vi "CRYGet Default Hardware.vi"(0 "Hardware Cluster In":T1={"Name"="", "Analog I/O"=0, "Digital I/O"=0, "Channels"=2, "Dig Dev ID"=1, "N ports"=3, "Interface"=0, "Dig I/O Ports"=[{"port #"=1, "width"=8, "direction"=0}, {"port #"=2, "width"=8, "direction"=0}, {"port #"=3, "width"=8, "direction"=0}], "Interf settings"=[], "N interfs"=3, "udev SNs"=[], "udev enable"=FALSE, "Channel Array"=[], "Cal sequence"="", "SelectedIn"=0, "SelectedOut"=0, "SelectedTab"=0, "State"=FALSE, "Help"="", "Advanced"=FALSE, "In Audio Driver"=0, "Out Audio Driver"=0} {"Channel Array"."Coupling" items=["Default"=-1, "RSE"=10083, "NRSE"=10078, "Differential"=10106, "Pseudodifferential"=12529]; "Channel Array"."term config" items=["Default"=-1, "RSE"=10083, "NRSE"=10078, "Differential"=10106, "Pseudodifferential"=12529]; "Channel Array"."Anti-aliasing Factor (%fs)" format="%.2f"}) -> (6 "I_Name Out":string[][](array[string]), 8 "O_Name Out":string[][](array[string]), 9 "Hardware Cluster Out":T1={"Name"="", "Analog I/O"=0, "Digital I/O"=0, "Channels"=2, "Dig Dev ID"=1, "N ports"=3, "Interface"=0, "Dig I/O Ports"=[{"port #"=1, "width"=8, "direction"=0}, {"port #"=2, "width"=8, "direction"=0}, {"port #"=3, "width"=8, "direction"=0}], "Interf settings"=[], "N interfs"=3, "udev SNs"=[], "udev enable"=FALSE, "Channel Array"=[], "Cal sequence"="", "SelectedIn"=0, "SelectedOut"=0, "SelectedTab"=0, "State"=FALSE, "Help"="", "Advanced"=FALSE, "In Audio Driver"=0, "Out Audio Driver"=0} {"Channel Array"."Coupling" items=["Default"=-1, "RSE"=10083, "NRSE"=10078, "Differential"=10106, "Pseudodifferential"=12529]; "Channel Array"."term config" items=["Default"=-1, "RSE"=10083, "NRSE"=10078, "Differential"=10106, "Pseudodifferential"=12529]; "Channel Array"."Anti-aliasing Factor (%fs)" format="%.2f"}, 10 "O_Device Info Out":T3(array[cluster]), 11 "AO_Hardware Channel Name Out":string[](array[string]), 12 "I_Device Info Out":T3(array[cluster]), 13 "AI_Hardware Channel Name Out":string[](array[string]), 14 "O_Channel Info Out":T2[](array[typedef]) {"Coupling" items=["Default"=-1, "RSE"=10083, "NRSE"=10078, "Differential"=10106, "Pseudodifferential"=12529]; "term config" items=["Default"=-1, "RSE"=10083, "NRSE"=10078, "Differential"=10106, "Pseudodifferential"=12529]; "Anti-aliasing Factor (%fs)" format="%.2f"}, 15 "I_Channel Info Out":T2[](array[typedef]) {"Coupling" items=["Default"=-1, "RSE"=10083, "NRSE"=10078, "Differential"=10106, "Pseudodifferential"=12529]; "term config" items=["Default"=-1, "RSE"=10083, "NRSE"=10078, "Differential"=10106, "Pseudodifferential"=12529]; "Anti-aliasing Factor (%fs)" format="%.2f"}, 16 "Real Output Device Name Out":cluster{"MME":string[], "ASIO":string[]}, 17 "Real Input Device Name Out":cluster{"MME":string[], "ASIO":string[]}, 18 "Error":bool, 19 "No Device Name":string[](array[string]))   [LabVIEW 2013]
uses:
  Typedef Control/CRYHardware Channel Info.ctl
  Typedef Control/CRYHardware.ctl
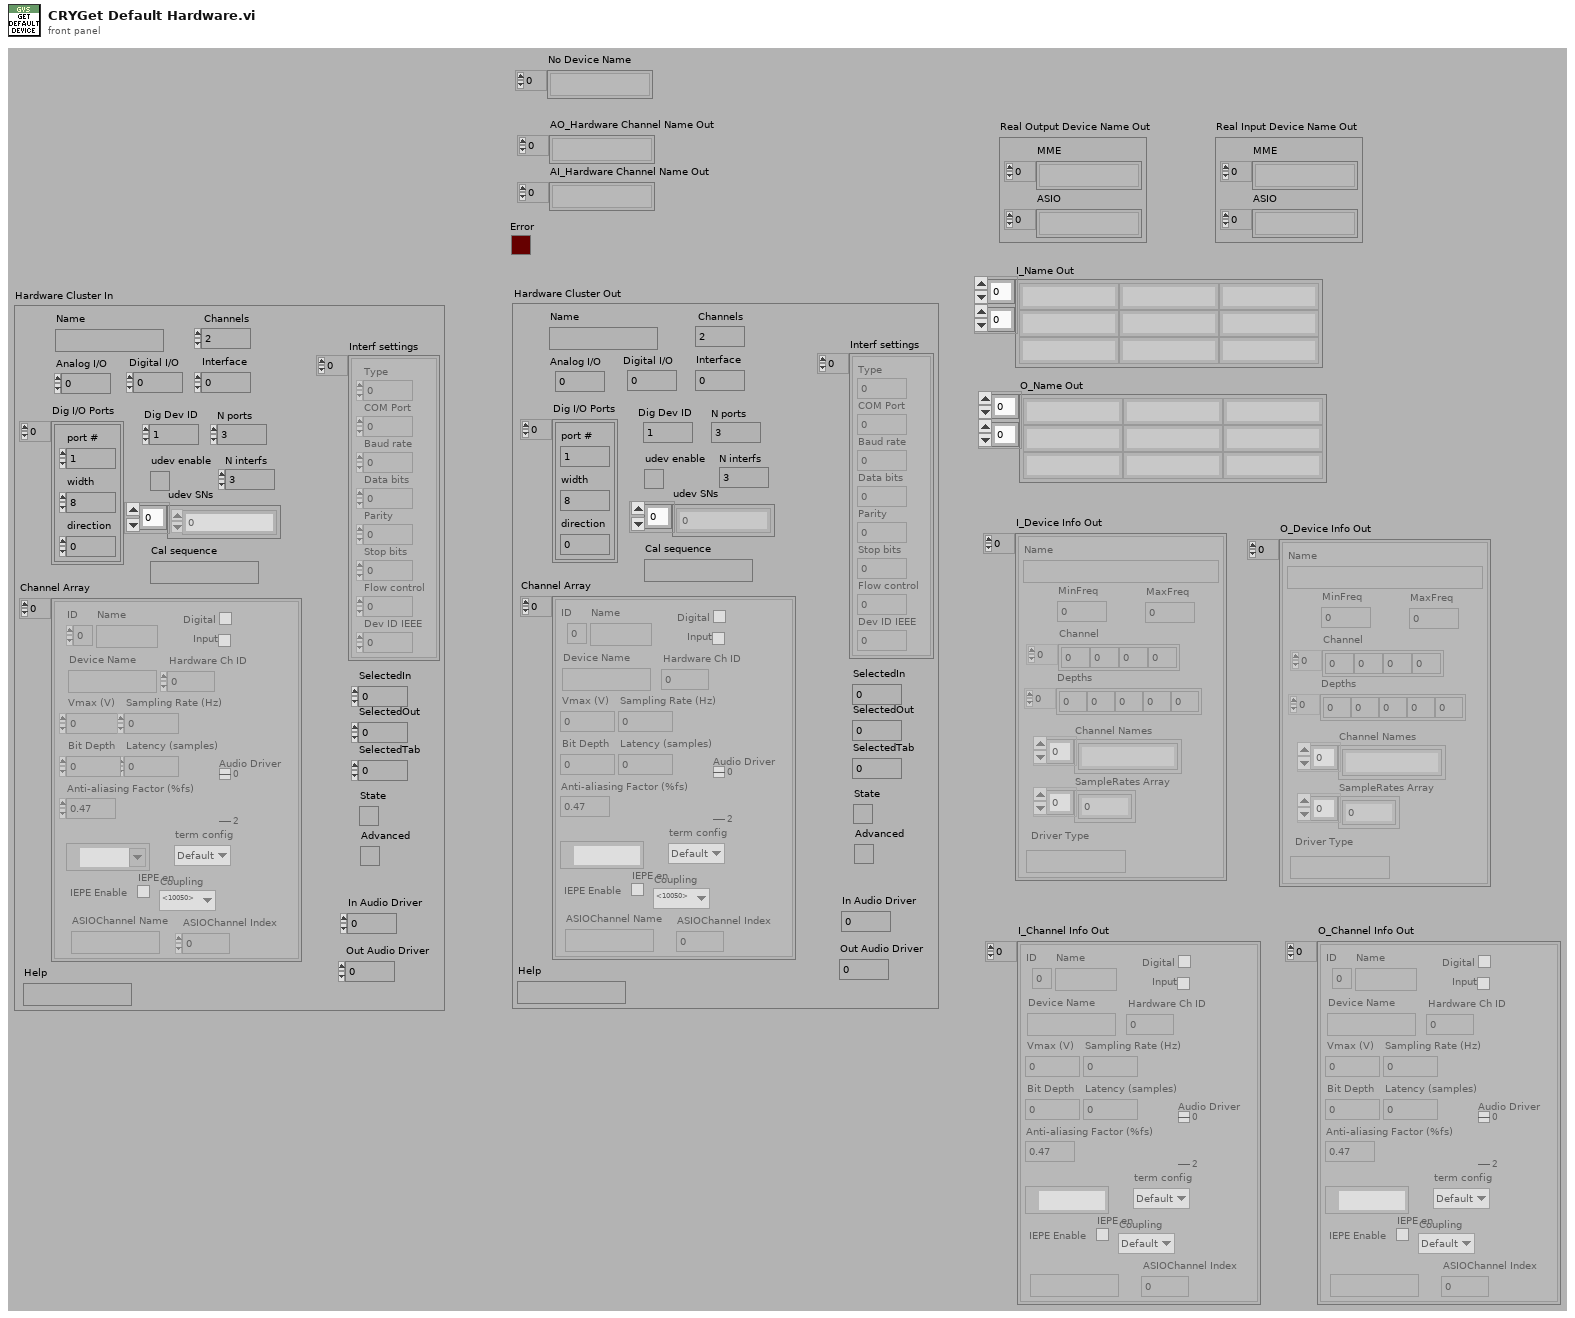
[diagram p1: front panel]
types:
  T1 = typedef "CRYHardware.ctl" = cluster{"Name":string, "Analog I/O":u16, "Digital I/O":u16, "Channels":u8, "Dig Dev ID":u8, "N ports":u8, "Interface":u32, "Dig I/O Ports":cluster{"port #":i16, "width":i16, "direction":i32}[], "Interf settings":cluster{"Type":u16, "COM Port":u8, "Baud rate":u32, "Data bits":u32, "Parity":u16, "Stop bits":u16, "Flow control":u16, "Dev ID IEEE":u8}[], "N interfs":i32, "udev SNs":i16[], "udev enable":bool, "Channel Array":T2[], "Cal sequence":string, "SelectedIn":u16, "SelectedOut":u16, "SelectedTab":u16, "State":bool, "Help":string, "Advanced":bool, "In Audio Driver":u16, "Out Audio Driver":u16}
  T2 = typedef "CRYHardware Channel Info.ctl" = cluster{"ID":i32, "Name":string, "Digital":bool, "Input":bool, "Device Name":string, "Hardware Ch ID":u8, "Vmax (V)":dbl, "Latency (samples)":dbl, "Sampling Rate (Hz)":u32, "Bit Depth":u32, "Anti-aliasing Factor (%fs)":sgl, "DAQmx Channel":tag, "term config":i32, "Coupling":i32, "IEPE en":bool, "ASIOChannel Name":string, "Audio Driver":u16, "ASIOChannel Index":u8}
  T3 = cluster{"Name":string, "MinFreq":dbl, "MaxFreq":dbl, "Channel":i32[], "Depths":i32[], "Channel Names":string[], "SampleRates Array":dbl[], "Driver Type":string}[]
  T4 = cluster{"Type":u16, "COM Port":u8, "Baud rate":u32, "Data bits":u32, "Parity":u16, "Stop bits":u16, "Flow control":u16, "Dev ID IEEE":u8}[]
  T5 = cluster{"port #":i16, "width":i16, "direction":i32}[]
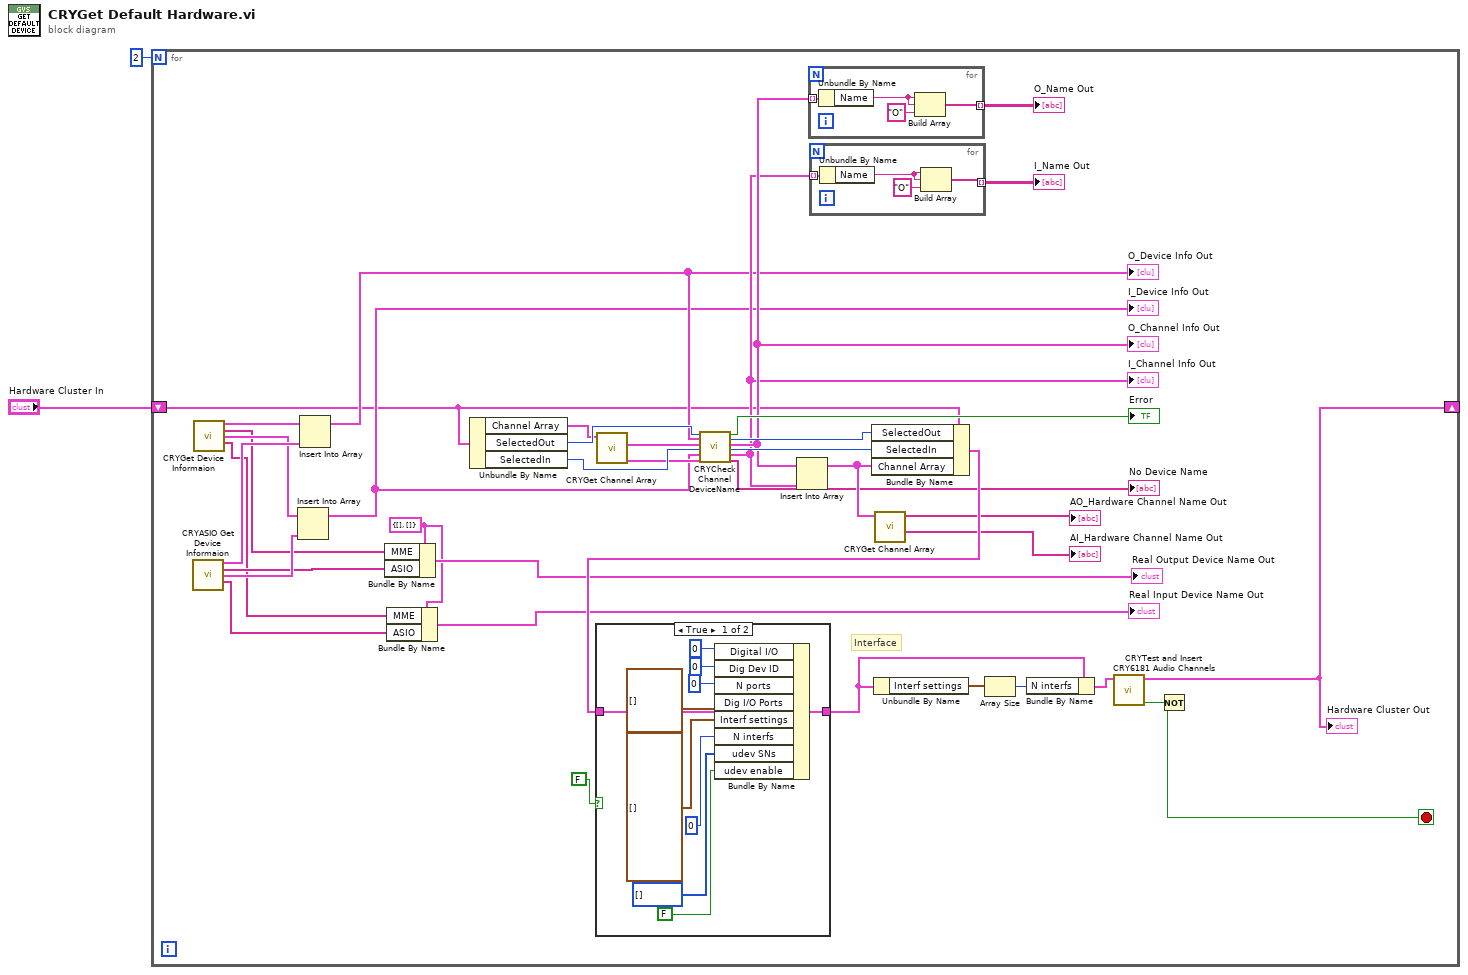
[diagram p0: block diagram]
diagram:
  n1 = for {
    N: 2 -> [_]
    shift-right: [w5] -> _
    shift-left: "Hardware Cluster In" -> [w9]
    stop <- w6 stop-if-true
    w13 = cluster{"MME":string[], "ASIO":string[]} {"MME"=[], "ASIO"=[]} ("Output Device Name Out")
    # "Interface"
    n2 = call "CRYASIO Get Device Informaion.vi"() -> ("ASIO Output Device Infor"=w22:T3, "ASIO Output Device Name"=w15:string[], "ASIO Input Device Infor"=w18:T3, "ASIO Input Device Name"=w10:string[])  [unwired: 11 in, 1 out]
    n3 = call "CRYGet Device Informaion.vi"() -> ("Output Device Infor"=w21:T3, "Output Device Name"=w16:string[], "Input Device Infor"=w19:T3, "Input Device Name"=w11:string[])  [unwired: 11 in, 1 out]
    n4 = Insert Into Array(array=w19, new element=w18) -> (w17:T3)  [unwired: 1 in]
    "I_Device Info Out" <- w17
    n5 = Insert Into Array(array=w21, new element=w22) -> (w20:T3)  [unwired: 1 in]
    "O_Device Info Out" <- w20
    n6 = Bundle By Name(cluster=w13, "MME"=w16, "ASIO"=w15) -> (→"Real Output Device Name Out":cluster{"MME":string[], "ASIO":string[]})
    n7 = Bundle By Name(cluster=w13, "MME"=w11, "ASIO"=w10) -> (→"Real Input Device Name Out":cluster{"MME":string[], "ASIO":string[]})
    n8 = Unbundle By Name(w9) -> ("Channel Array"=w32:T2[], "SelectedOut"=w40:u16, "SelectedIn"=w41:u16)
    n9 = call "CRYGet Channel Array.vi"("Channel Array"=w32) -> ("I Channel Info Out"=w36:T2[], "O Channel Info Out"=w35:T2[])  [unwired: 9 out]
    n10 = call "CRYCheck Channel DeviceName.vi"("SelectedOut"=w40, "O Device Info"=w20, "O Channel Info"=w35, "SelectedIn"=w41, "I Device Info"=w17, "I Channel Info"=w36) -> ("Check State"=→"Error":bool, "O SelectedN Out"=w37:u16, "O Channel Info Out"=w27:T2[], "I SelectedN Out"=w38:u16, "I Channel Info Out"=w26:T2[], "No Device Name"=→"No Device Name":string[])  [unwired: 8 out]
    "I_Channel Info Out" <- w26
    "O_Channel Info Out" <- w27
    n11 = Insert Into Array(array=w27, new element=w26) -> (w39:T2[])  [unwired: 1 in]
    n12 = for {
      tunnel: w27 -> [w49] mode=indexing
      tunnel: [w46] -> w23 mode=indexing
      n13 = Unbundle By Name(w49) -> ("Name"=w48:string)
      n14 = Build Array(w48, w48, "O" ("element")) -> (w46:string[])
    }
    "O_Name Out" <- w23
    n15 = for {
      tunnel: w26 -> [w45] mode=indexing
      tunnel: [w42] -> w24 mode=indexing
      n16 = Unbundle By Name(w45) -> ("Name"=w43:string)
      n17 = Build Array(w43, w43, "O" ("element")) -> (w42:string[])
    }
    "I_Name Out" <- w24
    n18 = Bundle By Name(cluster=w9, "SelectedOut"=w37, "SelectedIn"=w38, "Channel Array"=w39) -> (w29:T1)
    n19 = case shown="True" FALSE {
      tunnel: w29 -> [w59 w60]
      tunnel: [w50 w60] -> w30
      frame True {
        n20 = Bundle By Name(cluster=w59, "Digital I/O"=u16 0, "Dig Dev ID"=u8 0, "N ports"=u8 0, "Dig I/O Ports"=T5 [], "Interf settings"=T4 [], "N interfs"=0, "udev SNs"=i16[] [], "udev enable"=FALSE) -> (w50:T1)
      }
      frame False {
      }
    }
    n21 = Unbundle By Name(w30) -> ("Interf settings"=w33:T4)
    n22 = call "CRYGet Channel Array.vi"("Channel Array"=w39) -> ("I_Channel Name Out"=→"AI_Hardware Channel Name Out":string[], "O_Channel Name Out"=→"AO_Hardware Channel Name Out":string[])  [unwired: 9 out]
    n23 = Array Size(array=w33) -> (size(s)=w34:i32)
    n24 = Bundle By Name(cluster=w30, "N interfs"=w34) -> (w8:T1)
    n25 = call "CRYTest and Insert CRY6181 Audio Channels.vi"("Hardware in"=w8) -> ("Inserted channels"=w7:bool, "Hardware out"=w5:T1)  [unwired: 9 in]
    "Hardware Cluster Out" <- w5
    n26 = Not(x=w7) -> (.not. x?=w6:bool)
  }
